vi "QVA_ReadAttribute.vi"(0 "QueueIn":refnum<queue>, 2 "VariableName":string, 3 "Timeout [ms]":i32=-1, 5 "ErrorIn":errorcluster) -> (14 "QueueOut":refnum<queue>, 16 "ok":bool, 17 "Data":variant, 18 "Type":string, 19 "ErrorOut":errorcluster)   [LabVIEW 2016]
doc: "Liest eine Variable und den Datentypbeschrieb eines QVA aus\n\nsige / 3.12.13"
uses:
  private/QVA.VariableDataTypeDef.ctl
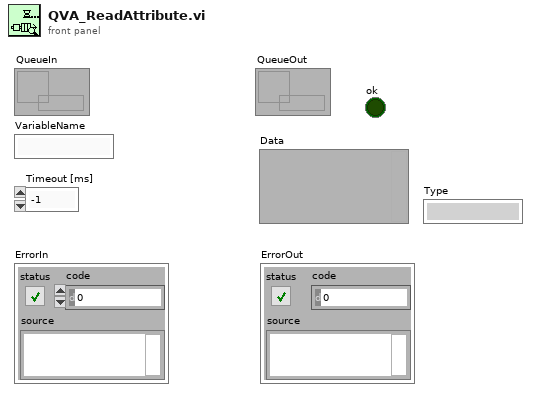
[diagram p1: front panel]
types:
  T1 = typedef "QVA.VariableDataTypeDef.ctl" = cluster{"Type":string, "Data":variant}
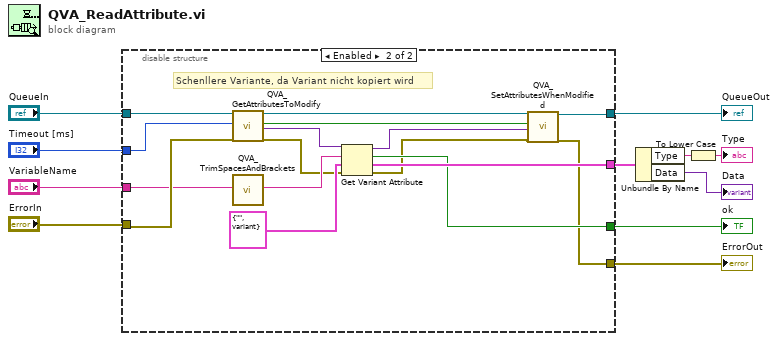
[diagram p0: block diagram]
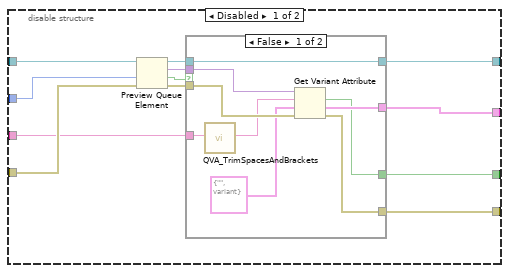
[diagram p2: hidden frame]
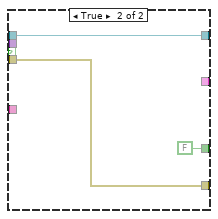
[diagram p3: hidden frame]
diagram:
  n1 = disable-structure shown="Enabled" {
    disable-tunnel: "ErrorIn" -> [w23 w48]
    disable-tunnel: "Timeout [ms]" -> [w22 w47]
    disable-tunnel: "QueueIn" -> [w21 w51]
    disable-tunnel: [w18 w38] -> w8
    disable-tunnel: [w17 w40] -> w7
    disable-tunnel: "VariableName" -> [w16 w43]
    disable-tunnel: [w15 w39] -> w3
    disable-tunnel: [w12 w49] -> w2
    frame Disabled {
      n2 = Preview Queue Element(queue=w21, timeout in ms (-1)=w22, error in (no error)=w23) -> (queue out=w13:refnum<queue>, element=w19:variant, timed out?=w14:bool, error out=w20:errorcluster)
      n3 = case shown="False" w14 {
        tunnel: w20 -> [w32 w34]
        tunnel: w19 -> [w31 _]
        tunnel: [w30 w34] -> w18
        tunnel: [w28 _] -> w17
        tunnel: w16 -> [w27 _]
        tunnel: [w26 FALSE] -> w15
        tunnel: w13 -> [w25 w35]
        tunnel: [w25 w35] -> w12
        frame False {
          n4 = call "QVA_TrimSpacesAndBrackets.vi"("String"=w27) -> ("TrimmedString"=w24:string)  [unwired: 18 in]
          n5 = Get Variant Attribute(Variant=w31, name=w24, default value (empty Variant)=T1 {"Type"="", "Data"=variant}, error in=w32) -> (found=w26:bool, value=w28:T1, error out=w30:errorcluster)  [unwired: 1 out]
        }
        frame True {
        }
      }
    }
    frame Enabled {
      # "Schenllere Variante, da Variant nicht kopiert wird"
      n6 = call "QVA_GetAttributesToModify.vi"("QueueIn"=w51, "Timeout"=w47, "ErrorIn"=w48) -> ("QueueOut"=w50:refnum<queue>, "Timeout"=w46:bool, "VariantData"=w45:variant, "ErrorOut"=w37:errorcluster)  [unwired: 13 in]
      n7 = call "QVA_TrimSpacesAndBrackets.vi"("String"=w43) -> ("TrimmedString"=w42:string)  [unwired: 18 in]
      n8 = Get Variant Attribute(Variant=w45, name=w42, default value (empty Variant)=T1 {"Type"="", "Data"=variant}, error in=w37) -> (duplicate Variant=w44:variant, found=w39:bool, value=w40:T1, error out=w36:errorcluster)
      n9 = call "QVA_SetAttributesWhenModified.vi"("QueueIn"=w50, "SkipAfterTimeout"=w46, "VariantData"=w44, "ErrorIn"=w36) -> ("QueueOut"=w49:refnum<queue>, "ErrorOut"=w38:errorcluster)  [unwired: 14 in]
    }
  }
  "QueueOut" <- w2
  "ErrorOut" <- w8
  "ok" <- w3
  n10 = Unbundle By Name(w7) -> ("Type"=w6:string, "Data"=→"Data":variant)
  n11 = To Lower Case(string=w6) -> (all lower case string=→"Type":string)
